vi "Inject Some Thangs.vi"(8 "error in (no error)":errorcluster, 9 "Attributes Ref":refnum<data-value>, 11 "Parallelizer in":refnum<class "Parallelizer.lvclass">) -> (0 "error out":errorcluster, 3 "Parallelizer out":refnum<class "Parallelizer.lvclass">)   [LabVIEW 2020, in "Test Executive.lvlib" / "Parallelizer Example.lvlib" / "Parallelizer.lvclass"]
uses:
  <vilib>/gpm_packages/@cs/test-executive/Source/Sandbox/Parallelizer Example/Parallelizer/Parallelizer.lvclass
  <vilib>/gpm_packages/@cs/lookup-table/Source/LookupTable/LookupTable.lvclass
  <vilib>/gpm_packages/@cs/lookup-table/Source/LookupTable/LookupTable.lvclass/LookupTable.ctl
  <vilib>/gpm_packages/@cs/test-executive/Source/Sandbox/Parallelizer Example/Parallelizer/Parallelizer.lvclass/Parallelizer.ctl
  b128af18-a1a8-4009-a015-da2cb315716f.vi
  <vilib>/gpm_packages/@cs/lookup-table/Source/LookupTable/Read Table Reference.vi
  b128af18-a1a8-4009-a015-da2cb315716f.vi/76a930fc-225c-4ff1-8a34-e59d4a2d9ddb.vi
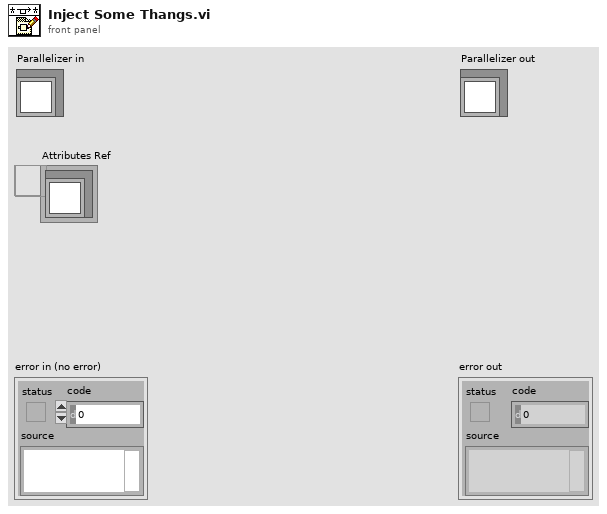
[diagram p1: front panel]
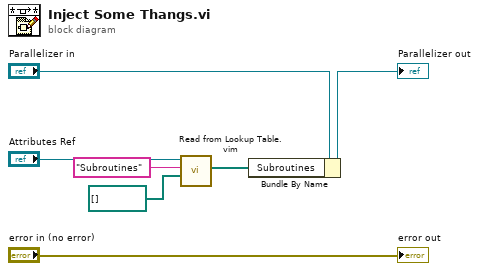
[diagram p0: block diagram]
diagram:
  n1 = call "Read from Lookup Table.vim"("Type"=path[] [], "Item Name"="Subroutines", "LookupTable Reference"="Attributes Ref") -> ("Value"=w3:path[])  [unwired: 5 in, 3 out]
  n2 = Bundle By Name(cluster="Parallelizer in", "Subroutines"=w3) -> (→"Parallelizer out":refnum<class "Parallelizer.lvclass">)
  "error out" <- "error in (no error)"
